vi "Voltage Level & Frequency.vi"(5 "Frequency Value (20.0 Hz)":dbl=20.0 min=20.0 max=30000000.0 step=1.0 format="%.4f", 7 "Current Level (0.0 A)":dbl min=0.0 max=0.2 step=0.01 format="%.4f", 8 "error in (no error)":errorcluster, 9 "Voltage Level (0.0 V)":dbl min=0.0 max=20.0 step=0.01 format="%.4f", 10 "Alc (F: Off)":bool, 11 "VISA resource name":refnum<visa-resource-name>) -> (0 "error out":errorcluster, 3 "VISA resource name out":refnum<visa-resource-name>)   [LabVIEW 2015, in "Agilent 428X Series.lvlib"]
doc: "This function sets the oscillator's output voltage/current level, frequency and switch ON/OFF Automatic Level Control (ALC)."
uses:
  Agilent 428X Series.lvlib
panel:
  # "On\nOff"
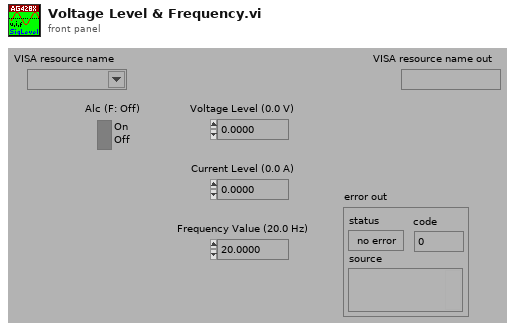
[diagram p1: front panel]
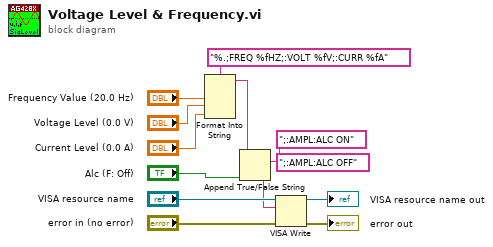
[diagram p0: block diagram]
diagram:
  n1 = Format Into String(format string="%.;FREQ %fHZ;:VOLT %fV;:CURR %fA", "Frequency Value (20.0 Hz)", "Voltage Level (0.0 V)", "Current Level (0.0 A)") -> (resulting string=w8:string)  [unwired: 2 in, 1 out]
  n2 = Append True/False String(1:"Alc (F: Off)", 2:";:AMPL:ALC OFF" ("true string"), 3:";:AMPL:ALC ON" ("true string"), 4:w8) -> (0:w1:string)
  n3 = VISA Write(VISA resource name="VISA resource name", write buffer=w1, error in (no error)="error in (no error)") -> (VISA resource name out=→"VISA resource name out":refnum<visa-resource-name>, error out=→"error out":errorcluster)  [unwired: 1 out]
